vi "Configure Arm.vi"(0 "VISA resource name":refnum<visa-resource-name>, 1 "Enable Arm Bypass (F: Disable)":bool, 5 "Arm Source (0: Immediate)":u16(ring) items=["Immediate", "Timer", "Bus", "Tlink", "Manual", "Negative SOT", "Positive SOT", "Bidirectional SOT"], 7 "Arm Loop Count (1)":i32=1, 9 "Arm Timer Interval (0.1 s)":dbl=0.1, 11 "error in (no error)":errorcluster) -> (4 "VISA resource name out":refnum<visa-resource-name>, 15 "error out":errorcluster)   [LabVIEW 2024, in "Keithley 648X Series.lvlib"]
doc: "Configures the event detection of the arm layer.\n\n<b>Note:</b>\nThis VI is part of the component handler interfacing VIs."
uses:
  <instrlib>/Keithley 648X Series/Keithley 648X Series.lvlib
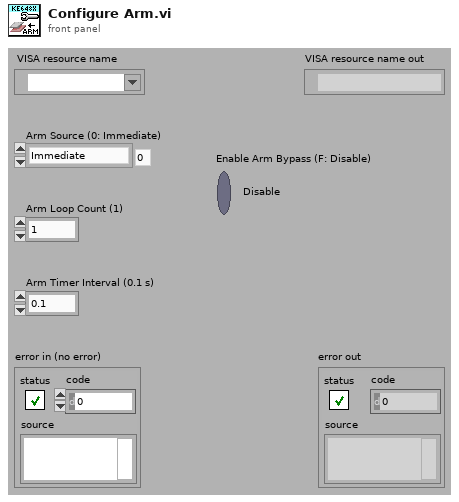
[diagram p1: front panel]
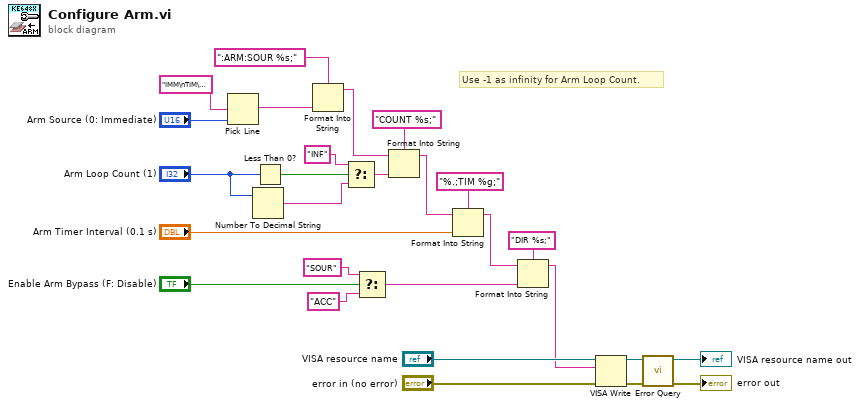
[diagram p0: block diagram]
diagram:
  # "Use -1 as infinity for Arm Loop Count."
  n1 = Pick Line(multi-line string="IMM\nTIM\nBUS\nTLIN\nMAN\nPST\nNST\nBST", line index="Arm Source (0: Immediate)") -> (output string=w19:string)  [unwired: 1 in]
  n2 = Number To Decimal String(number="Arm Loop Count (1)") -> (decimal integer string=w14:string)  [unwired: 1 in]
  n3 = Less Than 0?(x="Arm Loop Count (1)") -> (x < 0?=w16:bool)
  n4 = Format Into String(format string=":ARM:SOUR %s;", w19) -> (resulting string=w12:string)  [unwired: 2 in, 1 out]
  n5 = Select(t="INF", s=w16, f=w14) -> (s? t:f=w17:string)
  n6 = Select(t="SOUR", s="Enable Arm Bypass (F: Disable)", f="ACC" ("t")) -> (s? t:f=w5:string)
  n7 = Format Into String(format string="COUNT %s;", initial string=w12, w17) -> (resulting string=w9:string)  [unwired: 1 in, 1 out]
  n8 = Format Into String(format string="%.;TIM %g;", initial string=w9, "Arm Timer Interval (0.1 s)") -> (resulting string=w2:string)  [unwired: 1 in, 1 out]
  n9 = Format Into String(format string="DIR %s;", initial string=w2, w5) -> (resulting string=w1:string)  [unwired: 1 in, 1 out]
  n10 = VISA Write(VISA resource name="VISA resource name", write buffer=w1, error in (no error)="error in (no error)") -> (VISA resource name out=w23:refnum<visa-resource-name>, error out=w22:errorcluster)  [unwired: 1 out]
  n11 = call <instrlib>:"Error Query.vi"("error in (no error)"=w22, "VISA resource name"=w23) -> ("error out"=→"error out":errorcluster, "VISA resource name out"=→"VISA resource name out":refnum<visa-resource-name>)  [unwired: 6 in, 2 out]
